vi "Status Update.vi"(0 "Base Station":string, 1 "Status Reference":refnum<vi>, 5 "Band":string, 7 "Status":string, 9 "Value":string, 11 "error in (no error)":errorcluster) -> (15 "value out":errorcluster)   [LabVIEW 2021]
uses:
  aebbf0ec-7972-48c6-9654-a75ab60e4797.vi
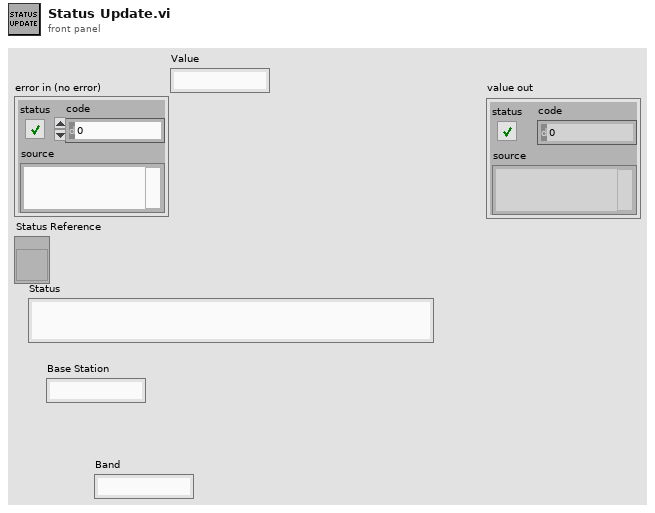
[diagram p1: front panel]
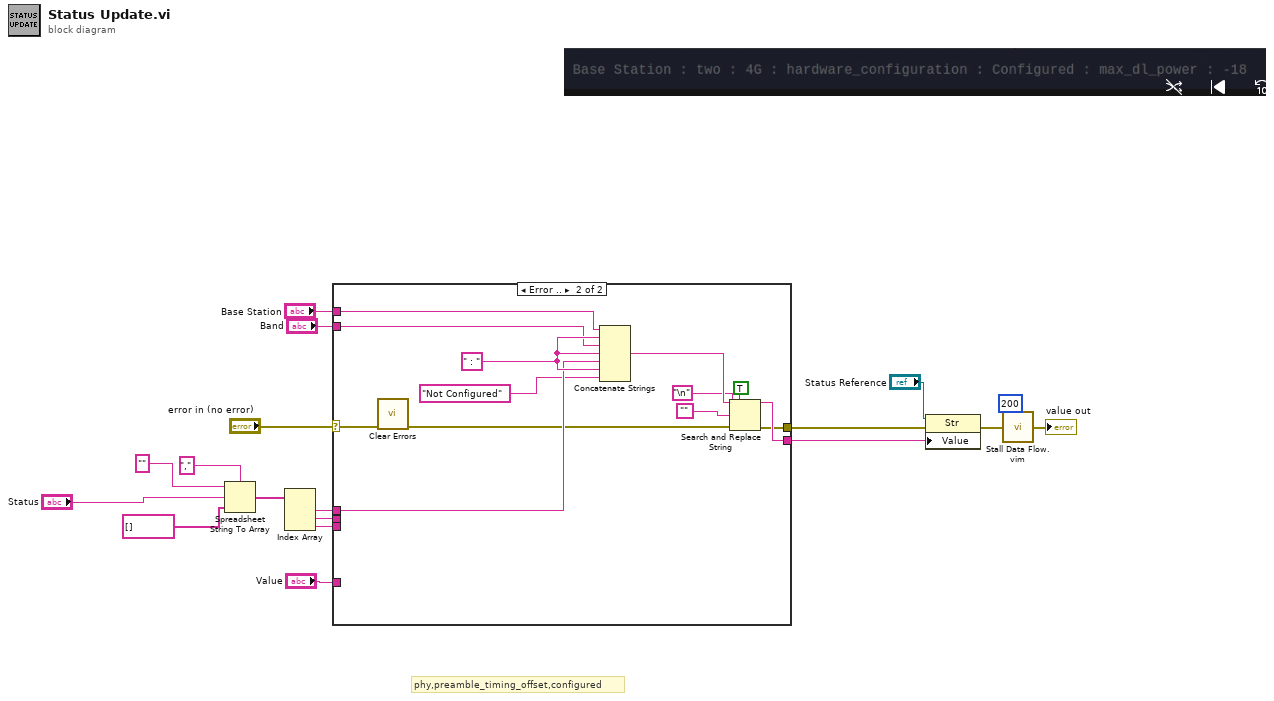
[diagram p0: block diagram]
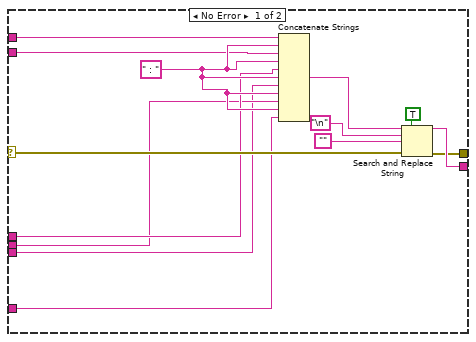
[diagram p2: hidden frame]
diagram:
  # "phy,preamble_timing_offset,configured"
  n1 = Spreadsheet String To Array(delimiter (Tab)=",", format string="", spreadsheet string="Status", array type (2D Dbl)=string[] [] ("Status 2")) -> (array=w7:string[])
  n2 = Index Array(array=w7) -> (element #1=w3:string, element #2=w2:string, element #3=w1:string)  [unwired: 3 in]
  n3 = case shown="Error .." "error in (no error)" {
    selector: "error in (no error)" -> [w26 w34]
    tunnel: [w27 w40] -> w13
    tunnel: [w25 w35] -> w12
    tunnel: "Band" -> [w24 w38]
    tunnel: "Base Station" -> [w23 w39]
    tunnel: "Value" -> [w22 _]
    tunnel: w3 -> [w21 w37]
    tunnel: w2 -> [w20 _]
    tunnel: w1 -> [w19 _]
    frame No Error {
      w32 = " : " ("delimiter (Tab)")
      n4 = Concatenate Strings(w23, w32, w24, w32, w21, w32, w19, w32, w20, w32, w22) -> (w31:string)
      n5 = Search and Replace String(replace all?=TRUE ("replace all? (F)"), input string=w31, search string="\n", replace string="", error in=w26) -> (result string=w27:string, error out=w25:errorcluster)  [unwired: 3 in, 2 out]
    }
    frame Error {
      w45 = " : " ("delimiter (Tab)")
      n6 = call <vilib>:"Clear Errors.vi"("error in (no error)"=w34) -> ("error out"=w33:errorcluster)  [unwired: 5 in, 1 out]
      n7 = Concatenate Strings(w39, w45, w38, w45, w37, w45, "Not Configured" ("string")) -> (w44:string)
      n8 = Search and Replace String(replace all?=TRUE ("replace all? (F)"), input string=w44, search string="\n", replace string="", error in=w33) -> (result string=w40:string, error out=w35:errorcluster)  [unwired: 3 in, 2 out]
    }
  }
  n9 = property class="Str"(reference="Status Reference", error in=w12, "Value"=w13) -> (error out=w17:errorcluster)  [unwired: 1 out]
  n10 = call "Stall Data Flow.vim"("value in"=w17, "milliseconds to wait"=u32 200) -> ("value out"=→"value out":errorcluster)  [unwired: 1 out]
